vi "RingValueFromString.vi"(8 "error in (no error)":errorcluster, 10 "String":string, 11 "Ring in":refnum<vi>) -> (0 "error out":errorcluster, 2 "Found":bool, 3 "Value":ext)   [LabVIEW 2013]
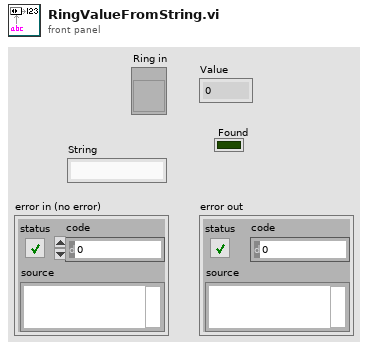
[diagram p1: front panel]
types:
  T1 = typedef "LVStringsAndValuesArrayTypeDef.ctl" = cluster{"String":string, "Value":ext}[]
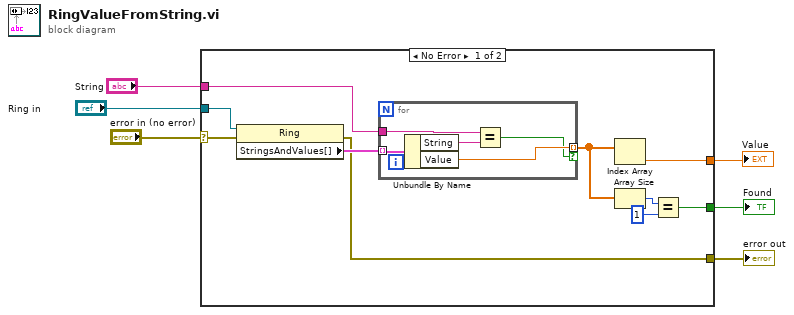
[diagram p0: block diagram]
diagram:
  n1 = case shown="No Error" "error in (no error)" {
    selector: "error in (no error)" -> [w8 w22]
    tunnel: "String" -> [w15 _]
    tunnel: "Ring in" -> [w14 _]
    tunnel: [w10 _] -> w3
    tunnel: [w9 _] -> w4
    tunnel: [w7 w22] -> w6
    frame No Error {
      n2 = property on="Property Node" class="Ring"(reference=w14, error in=w8) -> (error out=w7:errorcluster, "StringsAndValues[]"=w16:T1)  [unwired: 1 out]
      n3 = for {
        tunnel: w16 -> [w21] mode=indexing
        tunnel: w15 -> [w19]
        tunnel: [w18] -> w13 mode=indexing if=w17
        n4 = Unbundle By Name(w21) -> ("String"=w20:string, "Value"=w18:ext)
        n5 = Equal?(x=w19, y=w20) -> (x = y?=w17:bool)
      }
      n6 = Index Array(array=w13) -> (element=w9:ext)  [unwired: 1 in]
      n7 = Array Size(array=w13) -> (size(s)=w12:i32)
      n8 = Equal?(x=w12, y=1) -> (x = y?=w10:bool)
    }
    frame Error {
    }
  }
  "error out" <- w6
  "Value" <- w4
  "Found" <- w3
